vi "Get Data.vi"(8 "error in (no error)":errorcluster, 11 "TreeNode in":refnum<class "TreeNode.lvclass">) -> (0 "error out":errorcluster, 2 "Data out":refnum<class "Data.lvclass">, 3 "TreeNode out":refnum<class "TreeNode.lvclass">)   [LabVIEW 2013, in "MDSplus.lvlib" / "TreeNode.lvclass"]
doc: "Get Data for this node."
uses:
  <vilib>/MDSplus/Classes/Data_Class/TreeNode_Class/TreeNode.lvclass
  <vilib>/MDSplus/Classes/Data_Class/Data.lvclass
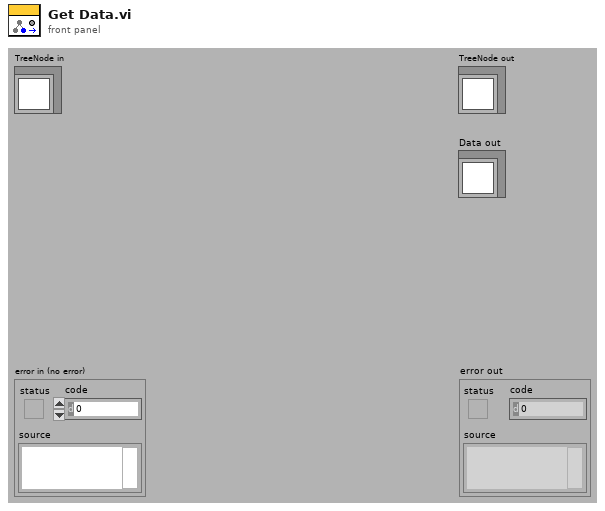
[diagram p1: front panel]
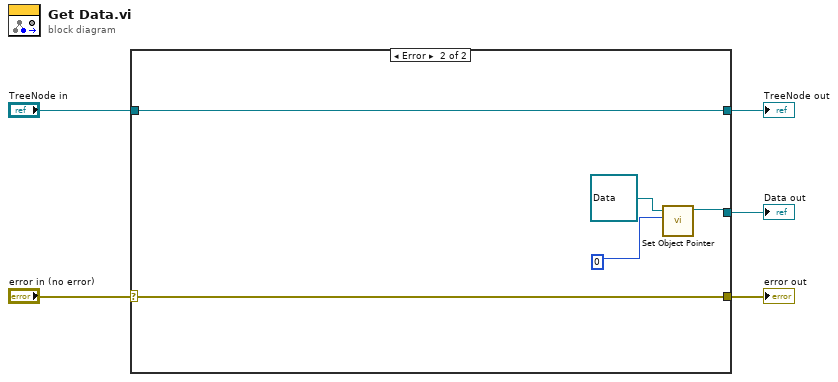
[diagram p0: block diagram]
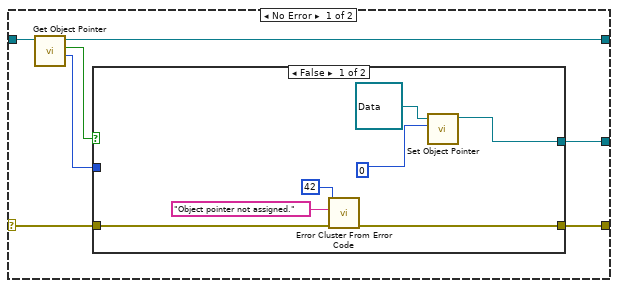
[diagram p2: hidden frame]
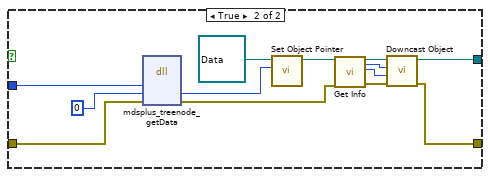
[diagram p3: hidden frame]
diagram:
  n1 = case shown="Error" "error in (no error)" {
    selector: "error in (no error)" -> [w8 w37]
    tunnel: [w7 w37] -> w4
    tunnel: [w6 w36] -> w2
    tunnel: "TreeNode in" -> [w11 w36]
    tunnel: [w12 w33] -> w1
    frame No Error {
      n2 = call-dynamic "Get Object Pointer.vi"("Data in"=w11) -> ("Object Pointer"=w9:i64, "Assigned object pointer?"=w10:bool, "Data out"=w6:refnum<class "TreeNode.lvclass">)  [unwired: 8 in]
      n3 = case shown="False" w10 {
        tunnel: [w13 w24] -> w12
        tunnel: w9 -> [_ w23]
        tunnel: w8 -> [w17 w21]
        tunnel: [w16 w20] -> w7
        frame False {
          n4 = call <vilib>:"Error Cluster From Error Code.vi"("error in (no error)"=w17, "error message (\"\")"="Object pointer not assigned." ("error message (\"\")"), "error code (0)"=42) -> ("error out"=w16:errorcluster)  [unwired: 6 in]
          n5 = call-dynamic "Set Object Pointer.vi"("Object Pointer"=0, "Data in"=refnum<class "Data.lvclass"> refnum ("Data out")) -> ("Data out"=w13:refnum<class "Data.lvclass">)  [unwired: 9 in]
        }
        frame True {
          n6 = dll-call lib="MDSobjectsLVShr" fn="mdsplus_treenode_getData"("lvTreeNodePtr"=w23, "lvDataPtrOut"=i64 0, "error"=w21) -> ("lvDataPtrOut"=w30:i64, "error"=w22:errorcluster)  [unwired: 5 in, 2 out]
          n7 = call-dynamic "Set Object Pointer.vi"("Object Pointer"=w30, "Data in"=refnum<class "Data.lvclass"> refnum ("Data.lvclass")) -> ("Data out"=w29:refnum<class "Data.lvclass">)  [unwired: 9 in]
          n8 = call-dynamic "Get Info.vi"("Data in"=w29, "error in (no error)"=w22) -> ("Data out"=w28:refnum<class "Data.lvclass">, "Class type out"=w27:u8, "Data type out"=w26:u8, "error out"=w25:errorcluster)  [unwired: 12 in, 2 out]
          n9 = call <vilib>:"Downcast Object.vi"("error in (no error)"=w25, "Data Type"=w26, "Class Type"=w27, "Data in"=w28) -> ("error out"=w20:errorcluster, "Data out"=w24:refnum<class "Data.lvclass">)  [unwired: 6 in]
        }
      }
    }
    frame Error {
      n10 = call-dynamic "Set Object Pointer.vi"("Object Pointer"=0, "Data in"=refnum<class "Data.lvclass"> refnum ("Data out")) -> ("Data out"=w33:refnum<class "Data.lvclass">)  [unwired: 9 in]
    }
  }
  "error out" <- w4
  "TreeNode out" <- w2
  "Data out" <- w1
